vi "KE6221 -- Get Arm Layer Trig Layer Wave Trig Params.vi"(0 "Resource In":refnum<visa-resource-name>, 1 "Check For SCPI Errors? (T)":bool=TRUE, 11 "error in (no error)":errorcluster) -> (4 "Resource Out (dupl)":refnum<visa-resource-name>, 8 "6221 Arm Trig Wave Trig Params":T1={"Arm Layer Input Trig Bypassed?"=FALSE, "Arm Layer Input Trig Source"=enum."Immediate", "Arm Layer Input Trig Link Line"=enum."1", "Arm Layer Input Trig Timer Interval (s)"=0.001, "Arm Layer Output Trig Mode"=enum."No Trig Out", "Arm Layer Output Trig Link Line"=enum."1", "Trig Layer Input Trig Source"=enum."Immediate", "Trig Layer Input Trig Link Line"=enum."1", "Trig Layer Output Trig Mode"=enum."No Trig Out", "Trig Layer Output Trig Link Line"=enum."1", "6221 Wave Input Trig Enabled?"=FALSE, "6221 Wave Input Trig Link Line"=enum."1", "6221 Wave Inactive Level (%)"=50.0, "6221 Wave Ingore Input Retrigs?"=FALSE, "6221 Phase Marker Output Trig Enabled?"=FALSE, "6221 Phase Marker (deg)"=180.0, "6221 Phase Marker Output Trig Link Line"=enum."1"} {"6221 Phase Marker (deg)" min=0.0 max=360.0 format="%.3f"; "6221 Wave Inactive Level (%)" min=-100.0 max=100.0 format="%.3p"; "Arm Layer Input Trig Timer Interval (s)" min=0.001 max=99999.999 step=0.001 format="%.3f"}, 15 "error out":errorcluster)   [LabVIEW 2019, in "Keithley 622x.lvlib"]
doc: "Returns the parameters for the 'Arm' and 'Trigger' layers of the trigger model, and also the trigger parameters for waveform playback. Note that this VI can only be used with the 6221, since the 6220 doesn't support waveform playback."
uses:
  Keithley 622x.lvlib
  Typedefs/KE6221 -- Arm Trig Wave Trig Params.ctl
  Low Level/Typedefs/KE622x -- Arm Source.ctl
  Low Level/Typedefs/KE622x -- Trig Link Line.ctl
  Low Level/Typedefs/KE622x -- Arm Timer Interval.ctl
  Low Level/Typedefs/KE622x -- Arm Output Mode.ctl
  Low Level/Typedefs/KE622x -- Trig Source.ctl
  Low Level/Typedefs/KE622x -- Trig Output Mode.ctl
  6221 Wave/Low Level/Typedefs/KE6221 -- Wave Extern Trig Link In Line.ctl
  6221 Wave/Low Level/Typedefs/KE6221 -- Wave Inactive Level.ctl
  6221 Wave/Low Level/Typedefs/KE6221 -- Wave Phase Marker.ctl
panel:
  # "Arm Layer"
  # "Trig Layer"
  # "KE6221 Wave"
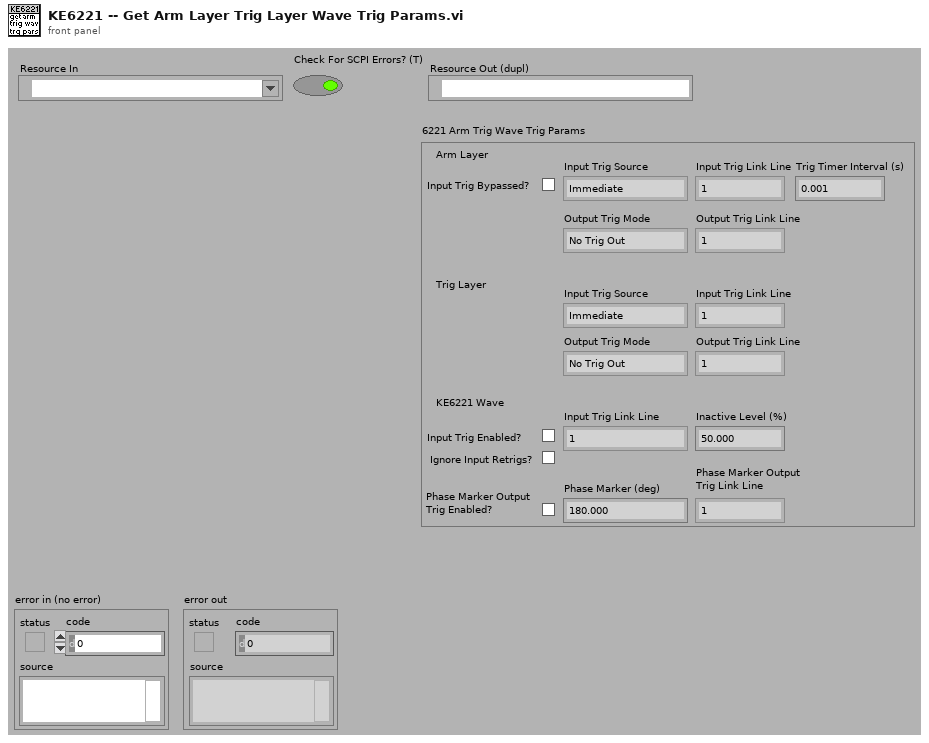
[diagram p1: front panel]
types:
  T1 = typedef "Keithley 622x.lvlib/KE6221 -- Arm Trig Wave Trig Params.ctl" = cluster{"Arm Layer Input Trig Bypassed?":bool, "Arm Layer Input Trig Source":T2, "Arm Layer Input Trig Link Line":T3, "Arm Layer Input Trig Timer Interval (s)":T4, "Arm Layer Output Trig Mode":T5, "Arm Layer Output Trig Link Line":T3, "Trig Layer Input Trig Source":T6, "Trig Layer Input Trig Link Line":T3, "Trig Layer Output Trig Mode":T7, "Trig Layer Output Trig Link Line":T3, "6221 Wave Input Trig Enabled?":bool, "6221 Wave Input Trig Link Line":T8, "6221 Wave Inactive Level (%)":T9, "6221 Wave Ingore Input Retrigs?":bool, "6221 Phase Marker Output Trig Enabled?":bool, "6221 Phase Marker (deg)":T10, "6221 Phase Marker Output Trig Link Line":T3}
  T2 = typedef "Keithley 622x.lvlib/KE622x -- Arm Source.ctl" = enum16{"Immediate", "Bus (*TRG)", "Timer", "Manual", "Trigger Link", "SOT Falling Edge", "SOT Rising Edge", "SOT Either Edge"}
  T3 = typedef "Keithley 622x.lvlib/KE622x -- Trig Link Line.ctl" = enum16{"1", "2", "3", "4", "5", "6"}
  T4 = typedef "Keithley 622x.lvlib/KE622x -- Arm Timer Interval.ctl" = dbl
  T5 = typedef "Keithley 622x.lvlib/KE622x -- Arm Output Mode.ctl" = enum16{"No Trig Out", "Trig Out On Enter Arm", "Trig Out On Exit Arm"}
  T6 = typedef "Keithley 622x.lvlib/KE622x -- Trig Source.ctl" = enum16{"Immediate", "Trigger Link"}
  T7 = typedef "Keithley 622x.lvlib/KE622x -- Trig Output Mode.ctl" = enum16{"No Trig Out", "Source Turn On", "After Source Delay"}
  T8 = typedef "Keithley 622x.lvlib/KE6221 -- Wave Extern Trig Link In Line.ctl" = enum16{"None", "1", "2", "3", "4", "5", "6"}
  T9 = typedef "Keithley 622x.lvlib/KE6221 -- Wave Inactive Level.ctl" = dbl
  T10 = typedef "Keithley 622x.lvlib/KE6221 -- Wave Phase Marker.ctl" = dbl
  T11 = typedef "Keithley 622x.lvlib/KE622x -- Arm Layer Params.ctl" = cluster{"Bypass Arm Layer\nInput Trigger?":bool, "Input Trig Source":T2, "Input Trig Link Line":T3, "Arm Timer Interval (s)":T4, "Output Trig Mode":T5, "Output Trig Link Line":T3}
  T12 = typedef "Keithley 622x.lvlib/KE622x -- Trig Layer Params.ctl" = cluster{"Input Trig Source":T6, "Input Trig Link Line":T3, "Output Trig Mode":T7, "Output Trig Link Line":T3}
  T13 = typedef "Keithley 622x.lvlib/KE6221 -- Wave External Trig Params.ctl" = cluster{"Ext Trig Enabled?":bool, "Trig Link In Line":T8, "Inactive Level (%)":T9, "Ignore Retrigs?":bool}
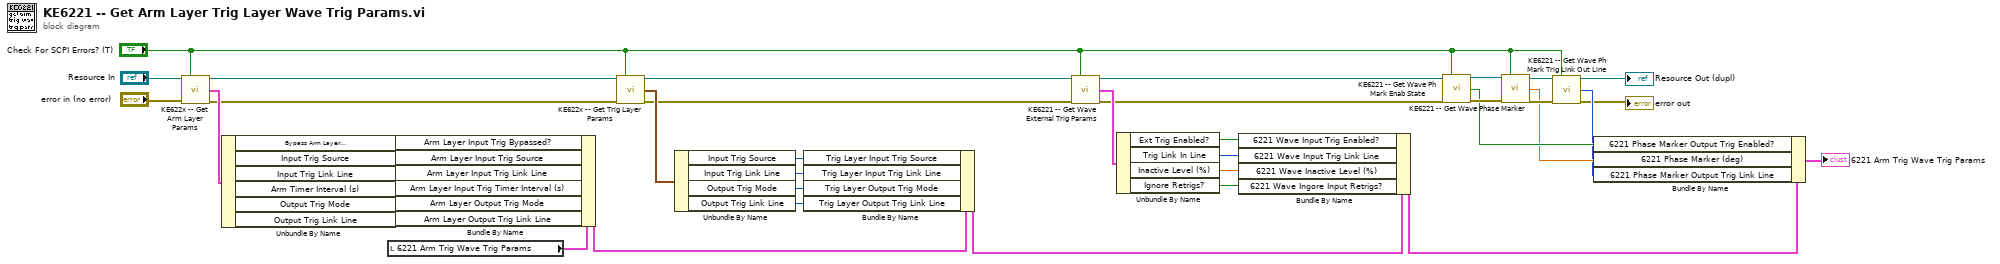
[diagram p0: block diagram]
diagram:
  n1 = call "KE622x -- Get Arm Layer Params.vi"("Resource In"="Resource In", "Check For SCPI Errors? (T)"="Check For SCPI Errors? (T)", "error in (no error)"="error in (no error)") -> ("Resource Out (dupl)"=w30:refnum<visa-resource-name>, "Arm Params"=w37:T11, "error out"=w29:errorcluster)  [unwired: 10 in]
  n2 = Unbundle By Name(w37) -> ("Bypass Arm Layer\nInput Trigger?"=w36:bool, "Input Trig Source"=w35:T2, "Input Trig Link Line"=w34:T3, "Arm Timer Interval (s)"=w33:T4, "Output Trig Mode"=w32:T5, "Output Trig Link Line"=w31:T3)
  n3 = local read "6221 Arm Trig Wave Trig Params"() -> (w38:T1)
  n4 = Bundle By Name(cluster=w38, "Arm Layer Input Trig Bypassed?"=w36, "Arm Layer Input Trig Source"=w35, "Arm Layer Input Trig Link Line"=w34, "Arm Layer Input Trig Timer Interval (s)"=w33, "Arm Layer Output Trig Mode"=w32, "Arm Layer Output Trig Link Line"=w31) -> (w28:T1)
  n5 = call "KE622x -- Get Trig Layer Params.vi"("Resource In"=w30, "Check For SCPI Errors? (T)"="Check For SCPI Errors? (T)", "error in (no error)"=w29) -> ("Resource Out (dupl)"=w22:refnum<visa-resource-name>, "Trig Layer Params"=w27:T12, "error out"=w21:errorcluster)  [unwired: 10 in]
  n6 = Unbundle By Name(w27) -> ("Input Trig Source"=w26:T6, "Input Trig Link Line"=w25:T3, "Output Trig Mode"=w24:T7, "Output Trig Link Line"=w23:T3)
  n7 = Bundle By Name(cluster=w28, "Trig Layer Input Trig Source"=w26, "Trig Layer Input Trig Link Line"=w25, "Trig Layer Output Trig Mode"=w24, "Trig Layer Output Trig Link Line"=w23) -> (w19:T1)
  n8 = call "KE6221 -- Get Wave External Trig Params.vi"("Resource In"=w22, "Check For SCPI Errors? (T)"="Check For SCPI Errors? (T)", "error in (no error)"=w21) -> ("Resource Out (dupl)"=w12:refnum<visa-resource-name>, "External Trig Params"=w20:T13, "error out"=w11:errorcluster)  [unwired: 10 in]
  n9 = Unbundle By Name(w20) -> ("Ext Trig Enabled?"=w18:bool, "Trig Link In Line"=w17:T8, "Inactive Level (%)"=w16:T9, "Ignore Retrigs?"=w15:bool)
  n10 = Bundle By Name(cluster=w19, "6221 Wave Input Trig Enabled?"=w18, "6221 Wave Input Trig Link Line"=w17, "6221 Wave Inactive Level (%)"=w16, "6221 Wave Ingore Input Retrigs?"=w15) -> (w7:T1)
  n11 = call "KE6221 -- Get Wave Ph Mark Enab State.vi"("Resource In"=w12, "Check For SCPI Errors? (T)"="Check For SCPI Errors? (T)", "error in (no error)"=w11) -> ("Resource Out (dupl)"=w10:refnum<visa-resource-name>, "Phase Marker Enabled?"=w8:bool, "error out"=w9:errorcluster)  [unwired: 10 in]
  n12 = call "KE6221 -- Get Wave Phase Marker.vi"("Resource In"=w10, "Check For SCPI Errors? (T)"="Check For SCPI Errors? (T)", "error in (no error)"=w9) -> ("Resource Out (dupl)"=w14:refnum<visa-resource-name>, "Phase Marker (deg)"=w6:T10, "error out"=w13:errorcluster)  [unwired: 10 in]
  n13 = call "KE6221 -- Get Wave Ph Mark Trig Link Out Line.vi"("Resource In"=w14, "Check For SCPI Errors? (T)"="Check For SCPI Errors? (T)", "error in (no error)"=w13) -> ("Resource Out (dupl)"=→"Resource Out (dupl)":refnum<visa-resource-name>, "Trig Link Out Line"=w5:T3, "error out"=→"error out":errorcluster)  [unwired: 10 in]
  n14 = Bundle By Name(cluster=w7, "6221 Phase Marker Output Trig Enabled?"=w8, "6221 Phase Marker (deg)"=w6, "6221 Phase Marker Output Trig Link Line"=w5) -> (→"6221 Arm Trig Wave Trig Params":T1)
